vi "Host Set Network.vi"() -> (0 "Reader":string, 3 "Writer":string)   [LabVIEW 2018]
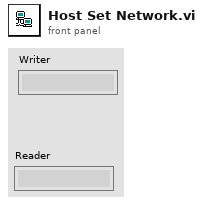
[diagram p1: front panel]
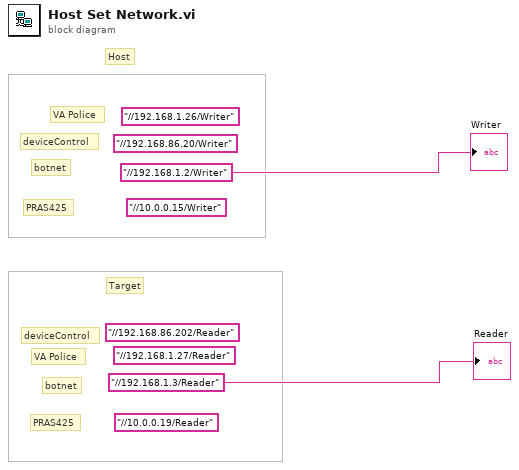
[diagram p0: block diagram]
diagram:
  (unwired) "//10.0.0.19/Reader" ("writer name")
  (unwired) "//10.0.0.15/Writer" ("writer name")
  (unwired) "//192.168.1.26/Writer" ("writer name")
  (unwired) "//192.168.1.27/Reader" ("reader url")
  (unwired) "//192.168.86.20/Writer" ("writer name")
  (unwired) "//192.168.86.202/Reader" ("reader url")
  # "PRAS425"
  # "PRAS425"
  # "botnet"
  # "botnet"
  # "deviceControl"
  # "deviceControl"
  # "VA Police"
  # "VA Police"
  # "Target"
  # "Host"
  "Writer" <- "//192.168.1.2/Writer" ("writer name")
  "Reader" <- "//192.168.1.3/Reader" ("reader url")
